vi "CSM Data Type String.vi"(10 "Data":variant) -> (2 "Data Type String":string)   [LabVIEW 2020, in "Communicable State Machine.lvlib"]
uses:
  Communicable State Machine.lvlib
  Data Type.ctl
  NI_Data Type.lvlib
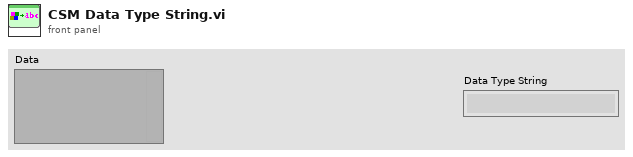
[diagram p1: front panel]
types:
  T1 = typedef "NI_Data Type.lvlib/Data Type.ctl" = enum8{"Invalid Type", "Void", "I8", "I16", "I32", "I64", "U8", "U16", "U32", "U64", "Single Float", "Double Float", "Extended Float", "Single Complex", "Double Complex", "Extended Complex", "Enum U8", "Enum U16", "Enum U32", "Enum U64", "Single Float With Unit", "Double Float With Unit", "Extended Float With Unit", "Single Complex with Unit", "Double Complex with Unit", "Extended Complex with Unit", "Boolean", "String", "Path", "Picture", "Tag", "Array", "Cluster", "Variant", "LV Variant", "Waveform", "Timestamp", "Digital Waveform", "Digital Data", "ExpressData", "Refnum", "External Data", "VI", "Poly VI", "LabVIEW Class Instance", "Fixed Point", "Set Collection", "Map Collection"}
  T2 = typedef "NI_Data Type.lvlib/Refnum Type.ctl" = enum16{"NotARefnum", "UnknownRefnum", "Generic", "Datalog", "ByteStream", "Device", "Occurence", "TCPNetConnection", "Auto", "Menu", "Imaq", "Hardware", "DataSocket", "Visa", "IVI", "UDPNetConnection", "Notifier", "Queue", "Irda", "EventReg", "DotNet", "UserEvent", "Callback", "UNUSED_EMPTY_POSITION", "BlueToothNetConnection", "LVObjApp", "LVObjVI", "LVObjUnknown", "GenericClass", "UserDefinedRefnumTag", "DataValue", "RT FIFO", "TDMS File", "PythonSessionRefnum"}
  T3 = typedef "NI_Data Type.lvlib/Tag Type.ctl" = enum16{"kNoTagType", "\tkDSCTagType", "\tkOldDAQTagType", "\tkIVITagType", "\tkVISATagType", "\tkGenClassTagType", "\tkUnusedTagType1", "\tkFPTagType", "\tkMotionTagType", "\tkDAQmxTaskTagType", "\tkDAQmxChannelTagType", "\tkDAQmxScaleTagType", "\tkDAQmxDeviceTagType", "\tkDAQmxTerminalTagType", "\tkDAQmxPhysChanTagType", "\tkDAQmxTriggerTagType", "\tkDAQmxSwitchTagType", "\tkDAQmxSignalTagType", "\tkUnusedTagType2", "\tkCANTaskTagType", "\tkCANInterfaceTagType", "\tkCANChannelTagType", "\tkNumTagTypes"}
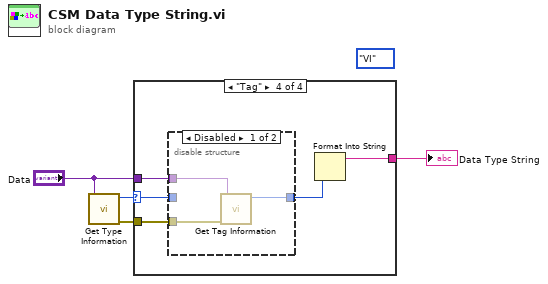
[diagram p0: block diagram]
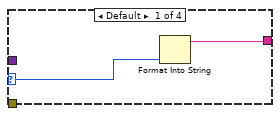
[diagram p2: hidden frame]
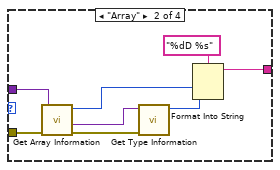
[diagram p3: hidden frame]
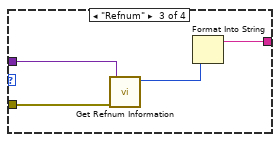
[diagram p4: hidden frame]
diagram:
  (unwired) Data_Type."VI" ("type")
  n1 = call "Get Type Information.vi"("variant"="Data") -> ("error out"=w3:errorcluster, "type"=w4:T1)  [unwired: 6 in, 3 out]
  n2 = case shown="\"Tag\"" w4 {
    selector: w4 -> [w5 _ _ w19]
    tunnel: w3 -> [_ w14 w18 w23]
    tunnel: "Data" -> [_ w13 w17 w22]
    tunnel: [w6 w7 w15 w20] -> w1
    frame Default {
      n3 = Format Into String(w5) -> (resulting string=w6:string)  [unwired: 3 in, 1 out]
    }
    frame "Array" {
      n4 = call "Get Array Information.vi"("error in (no error)"=w14, "variant"=w13) -> ("error out"=w12:errorcluster, "array element data type"=w9:variant, "number of dimensions"=w11:i32)  [unwired: 6 in, 1 out]
      n5 = call "Get Type Information.vi"("error in (no error)"=w12, "variant"=w9) -> ("type"=w8:T1)  [unwired: 5 in, 4 out]
      n6 = Format Into String(format string="%dD %s", w11, w8) -> (resulting string=w7:string)  [unwired: 2 in, 1 out]
    }
    frame "Refnum" {
      n7 = call "Get Refnum Information.vi"("error in (no error)"=w18, "variant"=w17) -> ("reference type"=w16:T2)  [unwired: 6 in, 3 out]
      n8 = Format Into String(w16) -> (resulting string=w15:string)  [unwired: 3 in, 1 out]
    }
    frame "Tag" {
      n9 = disable-structure shown="Disabled" {
        disable-tunnel: w23 -> [w26 _]
        disable-tunnel: w22 -> [w25 _]
        disable-tunnel: [w24 w27] -> w21
        disable-tunnel: w19 -> [_ w27]
        frame Disabled {
          n10 = call "Get Tag Information.vi"("error in (no error)"=w26, "variant"=w25) -> ("tag type"=w24:T3)  [unwired: 8 in, 1 out]
        }
        frame Enabled {
        }
      }
      n11 = Format Into String(w21) -> (resulting string=w20:string)  [unwired: 3 in, 1 out]
    }
  }
  "Data Type String" <- w1
